vi "Do.vi"(8 "error in (no error)":cluster{"状态":bool, "代码":i32, "源":string} caption="错误输入（无错误）", 10 "操作者输入":refnum<class "Actor.lvclass">, 11 "?":refnum<class "Update Water Level Msg.lvclass">) -> (0 "error out":cluster{"状态":bool, "代码":i32, "源":string} caption="错误输出", 2 "操作者输出":refnum<class "Actor.lvclass">)   [LabVIEW 2013, in "Evaporative Cooler Controller.lvlib" / "Update Water Level Msg.lvclass"]
uses:
  Update Water Level Msg.lvclass
  <vilib>/ActorFramework/Actor/Actor.lvclass
  Evaporative Cooler Controller/Evaporative Cooler Controller.lvclass
  Update Water Level Msg.lvclass/Update Water Level Msg.ctl
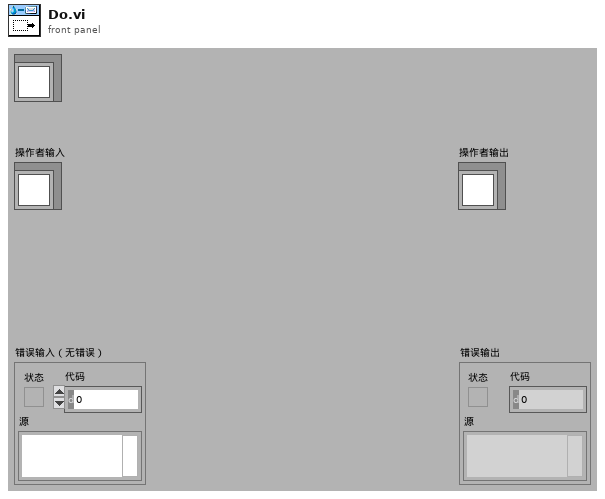
[diagram p1: front panel]
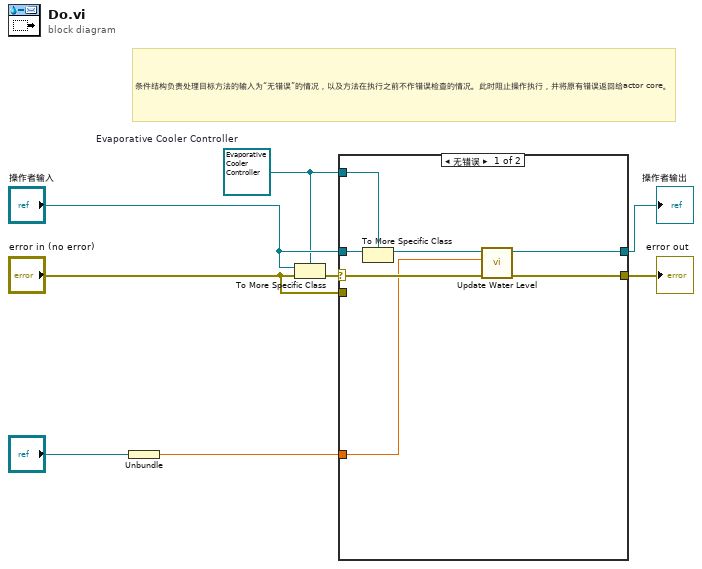
[diagram p0: block diagram]
diagram:
  w3 = refnum<class "Evaporative Cooler Controller.lvclass"> refnum  # Evaporative Cooler Controller
  # "条件结构负责处理目标方法的输入为“无错误”的情况，以及方法在执行之前不作错误检查的情况。此时阻止操作执行，并将原有错误返回给actor core。"
  n1 = Unbundle("?") -> (w2:dbl)
  n2 = To More Specific Class(target class=w3, reference="操作者输入", error in="error in (no error)") -> (error out=w7:errorcluster)  [unwired: 1 out]
  n3 = case shown="无错误" w7 {
    selector: w7 -> [w13 _]
    tunnel: [w15 w16] -> w6
    tunnel: [w14 w17] -> w5
    tunnel: "操作者输入" -> [w12 w17]
    tunnel: w3 -> [w11 _]
    tunnel: w2 -> [w9 _]
    tunnel: "error in (no error)" -> [_ w16]
    frame No Error {
      n4 = To More Specific Class(target class=w11, reference=w12) -> (specific class reference=w10:refnum<class "Evaporative Cooler Controller.lvclass">)  [unwired: 1 in, 1 out]
      n5 = call-dynamic "Update Water Level.vi"("error in (no error)"=w13, "水位"=w9, "蒸发冷却器的控制器输入"=w10) -> ("error out"=w15:cluster{"状态":bool, "代码":i32, "源":string}, "蒸发冷却器的控制器输出"=w14:refnum<class "Evaporative Cooler Controller.lvclass">)  [unwired: 7 in]
    }
    frame Error {
      # "该Do.vi与标准的Do.vi有点不同。此处如控制器的类型不正确也没有关系。如“转换为特定的类”函数输出错误，直接忽略该错误。这样做的好处是，蒸发冷却器能由普通的“冷却器的控制器”控制，即便普通的“冷却器的控制器” 无法处理蒸发冷却器的所有消息输出。由于输出的都是状态消息，可以不做特殊处理。"
    }
  }
  "error out" <- w6
  "操作者输出" <- w5
